vi "Configure Control AI Calib.vi"(0 "VISA resource name":refnum<visa-resource-name>, 1 "error in (no error)":errorcluster, 5 "Unit No. (0)":i32 min=0 max=6, 7 "Module No.(0)":i32 min=0 max=9, 9 "AI No.(1)":i32=1 min=1 max=2, 11 "Mode(0:Off)":i32 min=0 max=1, 12 "Number of Points":i32=2 min=2 max=12 step=1, 13 "Linearizar Points":cluster{"Input":i32, "Output":i32}[](array[cluster])) -> (4 "VISA resource name out":refnum<visa-resource-name>, 6 "Unit No.":i32, 8 "Module No.":i32, 10 "AI No.":i32, 15 "error out":errorcluster)   [LabVIEW 2020, in "Yokogawa GX Series.lvlib"]
doc: "Set input value correction of AI channel of PID module.\n\nCommand: SCtrlCalibAI"
uses:
  <instrlib>/Yokogawa GX Series/Yokogawa GX Series.lvlib
panel:
  in  "Correct Points":T1(array[cluster])
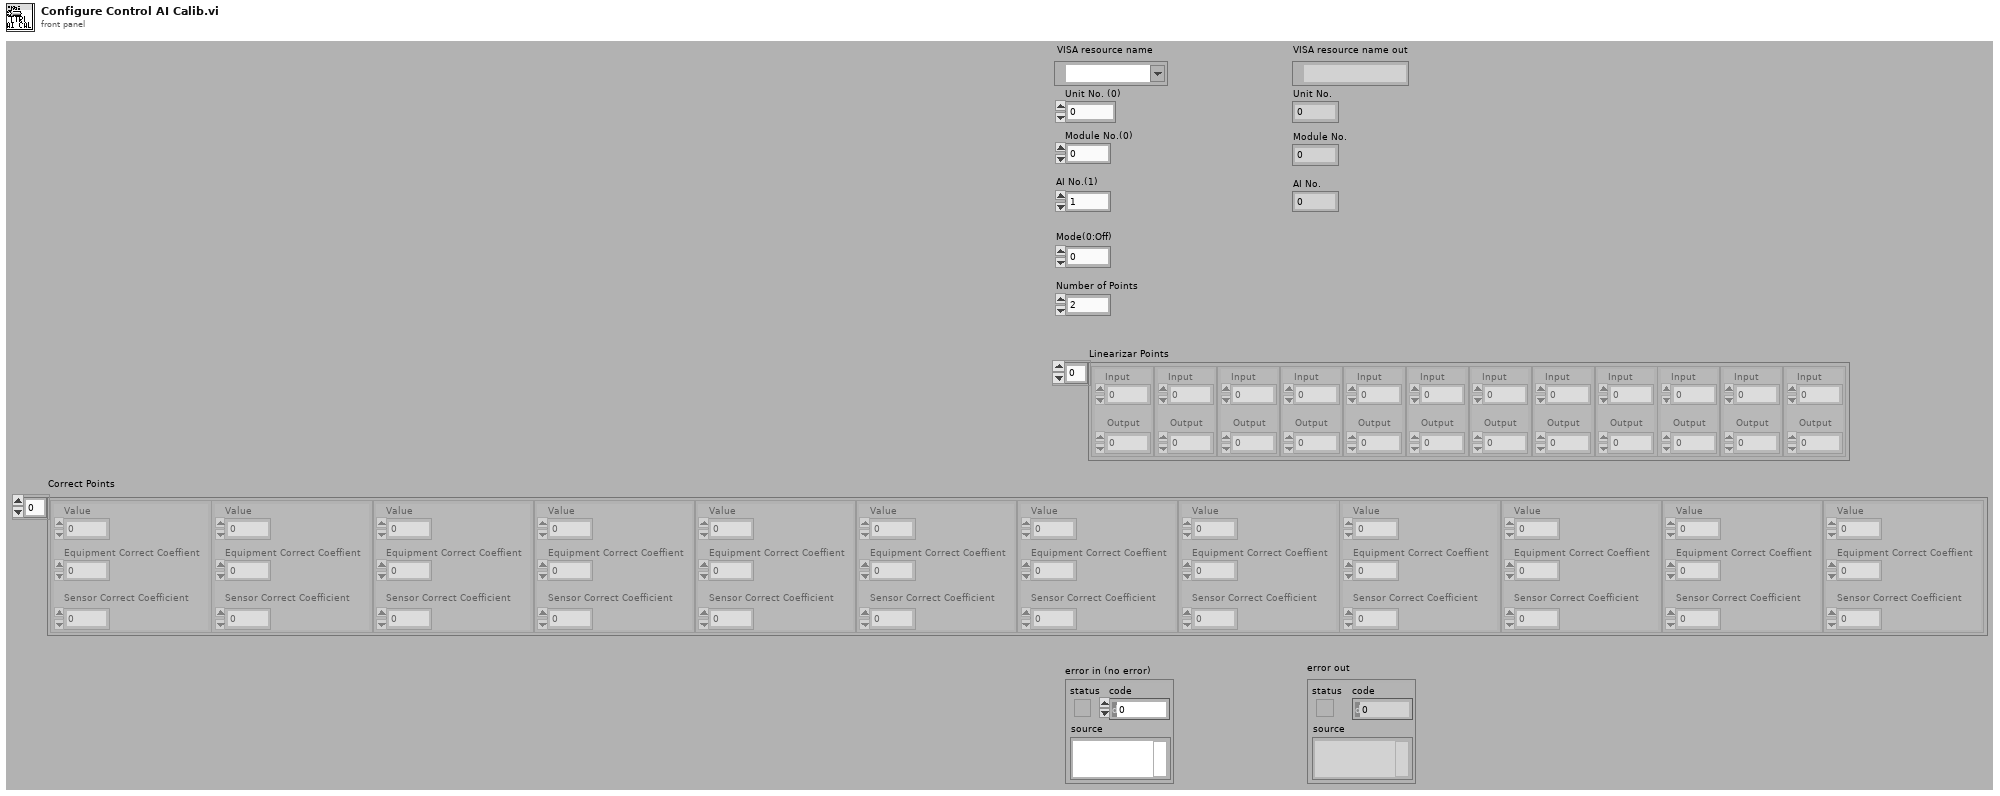
[diagram p1: front panel]
types:
  T1 = cluster{"Value":i32, "Equipment Correct Coeffient":i32, "Sensor Correct Coefficient":i32}[]
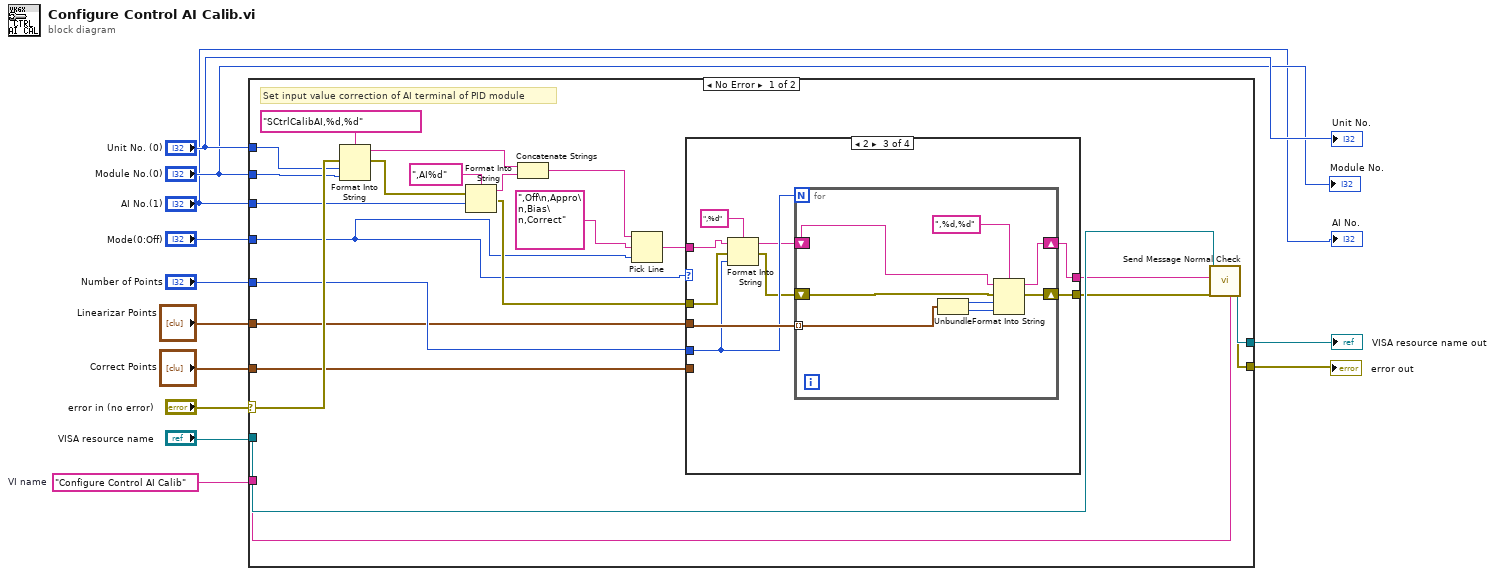
[diagram p0: block diagram]
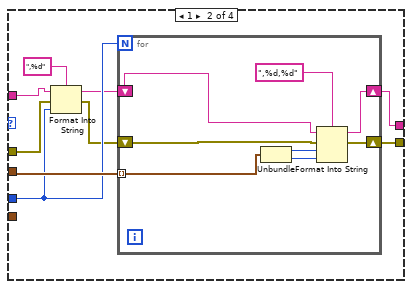
[diagram p3: hidden frame]
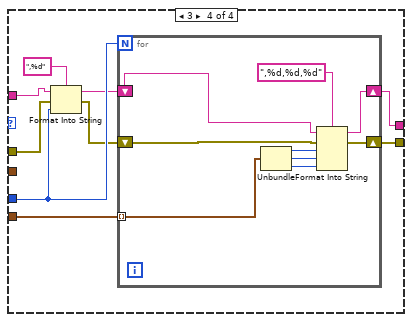
[diagram p4: hidden frame]
diagram:
  w8 = "Configure Control AI Calib"  # VI name
  n1 = case shown="No Error" "error in (no error)" {
    selector: "error in (no error)" -> [w31 w90]
    tunnel: [w35 w91] -> w12
    tunnel: [w34 w90] -> w11
    tunnel: "VISA resource name" -> [w33 w91]
    tunnel: w8 -> [w30 _]
    tunnel: "Unit No. (0)" -> [w29 _]
    tunnel: "Module No.(0)" -> [w28 _]
    tunnel: "AI No.(1)" -> [w26 _]
    tunnel: "Number of Points" -> [w19 _]
    tunnel: "Mode(0:Off)" -> [w14 _]
    tunnel: "Linearizar Points" -> [w18 _]
    tunnel: "Correct Points" -> [w13 _]
    frame No Error {
      # "Set input value correction of AI terminal of PID module"
      n2 = Format Into String(format string="SCtrlCalibAI,%d,%d", error in=w31, w29, w28) -> (resulting string=w24:string, error out=w25:errorcluster)  [unwired: 1 in]
      n3 = Format Into String(format string=",AI%d", error in=w25, w26) -> (resulting string=w23:string, error out=w17:errorcluster)  [unwired: 1 in]
      n4 = Concatenate Strings(w24, w23) -> (w22:string)
      n5 = Pick Line(string ("")=w22, multi-line string=",Off\n,Appro\n,Bias\n,Correct", line index=w14) -> (output string=w20:string)
      n6 = case shown="2" w14 {
        tunnel: [w37 w41 w58 w76] -> w16
        tunnel: w20 -> [w37 w44 w61 w79]
        tunnel: w19 -> [_ w43 w60 w78]
        tunnel: w18 -> [_ w46 w63 _]
        tunnel: w17 -> [w36 w40 w57 w75]
        tunnel: [w36 w38 w55 w73] -> w15
        tunnel: w13 -> [_ _ _ w72]
        frame 0, Default {
        }
        frame 1 {
          n7 = Format Into String(format string=",%d", initial string=w44, error in=w40, w43) -> (resulting string=w42:string, error out=w39:errorcluster)
          n8 = for {
            N: w43 -> [_]
            tunnel: w46 -> [w47] mode=indexing
            shift-right: [w50] -> w41
            shift-left: w42 -> [w51]
            shift-right: [w48] -> w38
            shift-left: w39 -> [w49]
            n9 = Unbundle(w47) -> ("Input"=w54:i32, "Output"=w53:i32)
            n10 = Format Into String(format string=",%d,%d", initial string=w51, error in=w49, w54, w53) -> (resulting string=w50:string, error out=w48:errorcluster)
          }
        }
        frame 2 {
          n11 = Format Into String(format string=",%d", initial string=w61, error in=w57, w60) -> (resulting string=w59:string, error out=w56:errorcluster)
          n12 = for {
            N: w60 -> [_]
            tunnel: w63 -> [w64] mode=indexing
            shift-right: [w67] -> w58
            shift-left: w59 -> [w68]
            shift-right: [w65] -> w55
            shift-left: w56 -> [w66]
            n13 = Unbundle(w64) -> ("Input"=w71:i32, "Output"=w70:i32)
            n14 = Format Into String(format string=",%d,%d", initial string=w68, error in=w66, w71, w70) -> (resulting string=w67:string, error out=w65:errorcluster)
          }
        }
        frame 3 {
          n15 = Format Into String(format string=",%d", initial string=w79, error in=w75, w78) -> (resulting string=w77:string, error out=w74:errorcluster)
          n16 = for {
            N: w78 -> [_]
            shift-right: [w85] -> w76
            shift-left: w77 -> [w86]
            shift-right: [w83] -> w73
            shift-left: w74 -> [w84]
            tunnel: w72 -> [w82] mode=indexing
            n17 = Unbundle(w82) -> ("Value"=w89:i32, "Equipment Correct Coeffient"=w88:i32, "Sensor Correct Coefficient"=w81:i32)
            n18 = Format Into String(format string=",%d,%d,%d", initial string=w86, error in=w84, w89, w88, w81) -> (resulting string=w85:string, error out=w83:errorcluster)
          }
        }
      }
      n19 = call <instrlib>:"Send Message Normal Check.vi"("Source (\"\")"=w30, "error in (no error)"=w15, "Send Message (\"\")"=w16, "VISA resource name"=w33) -> ("error out"=w34:errorcluster, "VISA resource name out"=w35:refnum<visa-resource-name>)  [unwired: 2 in, 4 out]
    }
    frame Error {
    }
  }
  "error out" <- w11
  "VISA resource name out" <- w12
  "Unit No." <- "Unit No. (0)"
  "Module No." <- "Module No.(0)"
  "AI No." <- "AI No.(1)"
